vi "Zadanie1.vi"() -> ()   [LabVIEW 2024]
panel:
  out "out":i32
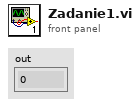
[diagram p1: front panel]
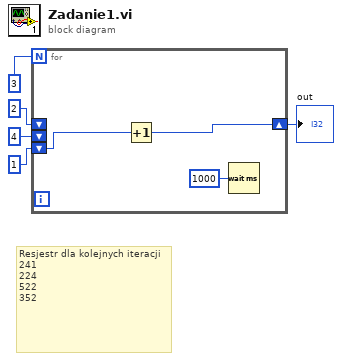
[diagram p0: block diagram]
diagram:
  # "Resjestr dla kolejnych iteracji\n241\n224\n522\n352"
  n1 = for {
    N: 3 -> [_]
    shift-right: [w6] -> w1
    shift-left: 2 -> [_]
    shift-left: 4 -> [_]
    shift-left: 1 -> [w8]
    n2 = Increment(x=w8) -> (x+1=w6:i32)
    n3 = Wait (ms)(milliseconds to wait=u32 1000) -> ()  [unwired: 1 out]
  }
  "out" <- w1
